vi "Save TS Results.vi"(8 "error in":errorcluster, 11 "Test Stand in":refnum<class "Generic Test Stand.lvclass">) -> (0 "error out":errorcluster, 3 "Test Stand out":refnum<class "Generic Test Stand.lvclass">)   [LabVIEW 2019, in "Generic Test Stand.lvclass"]
uses:
  Generic Test Stand.lvclass
  Generic Test Stand.lvclass/Generic Test Stand.ctl
  DAC/DAC.lvclass
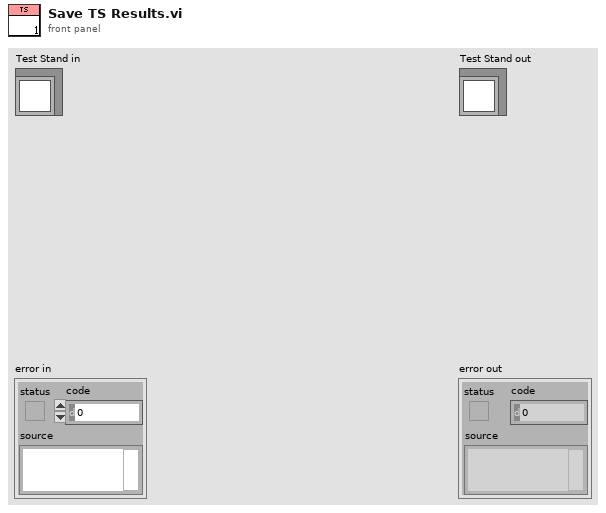
[diagram p1: front panel]
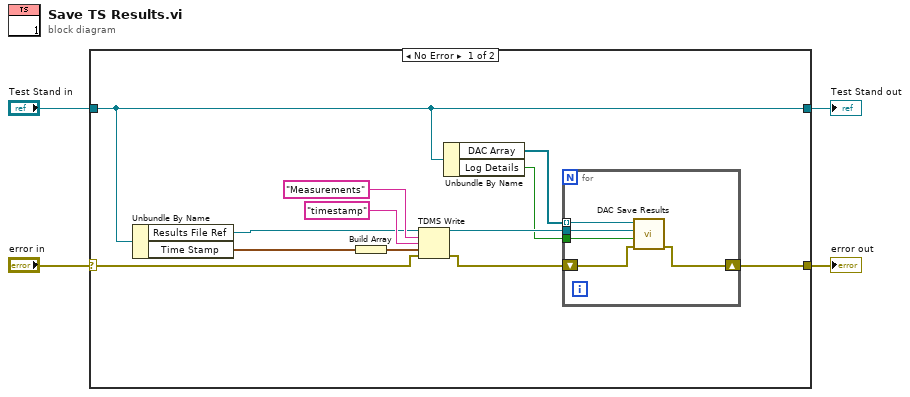
[diagram p0: block diagram]
diagram:
  n1 = case shown="No Error" "error in" {
    selector: "error in" -> [w6 w23]
    tunnel: [w5 w23] -> w3
    tunnel: [w11 w22] -> w1
    tunnel: "Test Stand in" -> [w11 w22]
    frame No Error {
      n2 = Unbundle By Name(w11) -> ("Results File Ref"=w8:refnum<k34>, "Time Stamp"=w7:timestamp)
      n3 = Build Array(w7) -> (w16:timestamp[])
      n4 = TDMS Write(0:w8, 5:"Measurements" ("group name in (Untitled)"), 7:"timestamp" ("group name in (Untitled)"), 9:w16, 11:w6) -> (4:w13:refnum<k34>, 15:w12:errorcluster)  [unwired: 1 in, 2 out]
      n5 = Unbundle By Name(w11) -> ("DAC Array"=w10:refnum<class "DAC.lvclass">[], "Log Details"=w9:bool)
      n6 = for {
        tunnel: w10 -> [w21] mode=indexing
        shift-right: [w18] -> w5
        shift-left: w12 -> [w19]
        tunnel: w13 -> [w20]
        tunnel: w9 -> [w17]
        n7 = call-dynamic "DAC Save Results.vi"("error in"=w19, "Log Details?"=w17, "tdms file"=w20, "DAC in"=w21) -> ("error out"=w18:errorcluster)  [unwired: 7 in]
      }
    }
    frame Error {
    }
  }
  "error out" <- w3
  "Test Stand out" <- w1
